vi "RTS Get Seq Index.vi"(8 "error in (no error)":errorcluster, 11 "Chamber 1-1 Input":T1[](array[typedef]) {"Start Time" format="%<%X\n%x>T"; "End Time" format="%<%X\n%x>T"}) -> (0 "Error Out":errorcluster, 1 "Times Up?":bool, 2 "Index Number":i32, 3 "Chamber 1-1 Output":T1[](array[typedef]) {"Start Time" format="%<%X\n%x>T"; "End Time" format="%<%X\n%x>T"})   [LabVIEW 2016]
uses:
  Type Definitions/RTS Door Ops Client.ctl
  Type Definitions/RTS Door Opening Schedule.ctl
  Type Definitions/RTS Door Ops Sequence.ctl
panel:
  # "Chamber Conditions:"
  # "Chamber Conditions:"
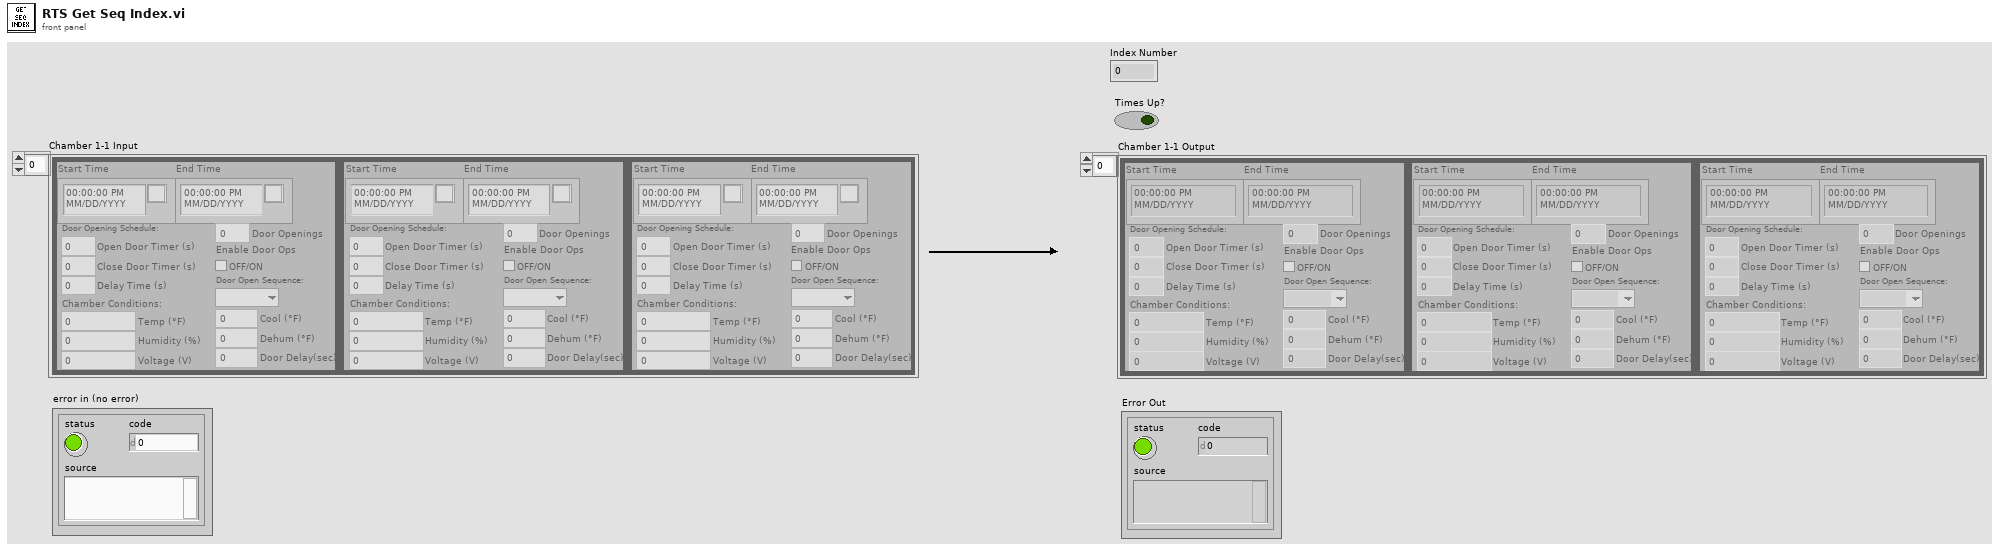
[diagram p1: front panel]
types:
  T1 = typedef "RTS Door Ops Client.ctl" = cluster{"End Time":timestamp, "Start Time":timestamp, "Door Opening Schedule:":T2, "Enable Door Ops":bool, "Door Openings":u32, "Temp (°F)":dbl, "Humidity (%)":dbl, "Voltage (V)":dbl, "Door Open Sequence:":T3, "Door Delay(sec)":dbl, "Dehum (°F)":dbl, "Cool (°F)":dbl}
  T2 = typedef "RTS Door Opening Schedule.ctl" = cluster{"Open Door Timer (s)":dbl, "Delay Time (s)":dbl, "Close Door Timer (s)":dbl}
  T3 = typedef "RTS Door Ops Sequence.ctl" = enum16{"", "1st", "2nd", "3rd"}
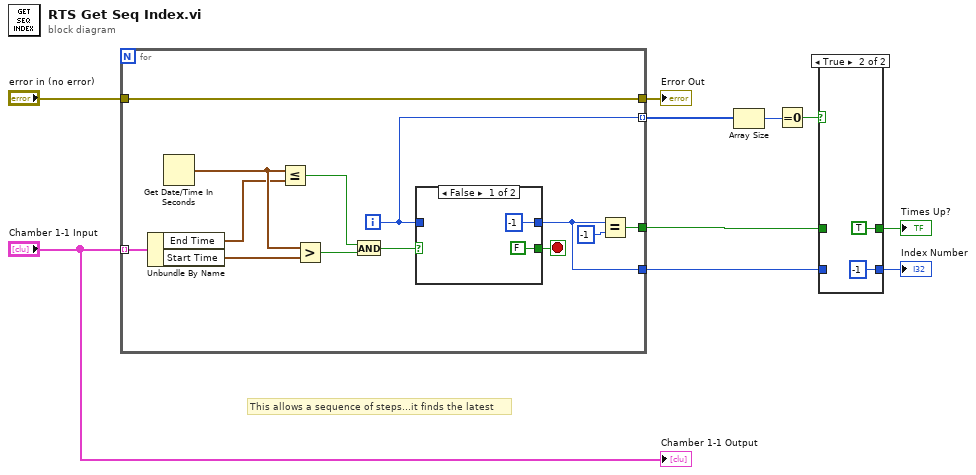
[diagram p0: block diagram]
diagram:
  # "This allows a sequence of steps...it finds the latest"
  n1 = for {
    tunnel: [w22] -> w7
    tunnel: "Chamber 1-1 Input" -> [w16] mode=indexing
    tunnel: [w13] -> w9
    tunnel: "error in (no error)" -> [w15]
    tunnel: [w15] -> w6
    tunnel: [w11] -> w5 mode=indexing
    i -> [w11]
    stop <- w12 stop-if-true
    n2 = Unbundle By Name(w16) -> ("End Time"=w14:timestamp, "Start Time"=w18:timestamp)
    n3 = Get Date/Time In Seconds() -> (seconds since 1Jan1904=w19:timestamp)
    n4 = Less Or Equal?(x=w19, y=w14) -> (x <= y?=w21:bool)
    n5 = Greater?(x=w19, y=w18) -> (0:w20:bool)
    n6 = And(x=w21, y=w20) -> (x .and. y?=w17:bool)
    n7 = case shown="False" w17 {
      selector: w17 -> [_ w26]
      tunnel: [-1 w27] -> w13
      tunnel: w11 -> [_ w27]
      tunnel: [FALSE w26] -> w12
      frame False {
      }
      frame True {
      }
    }
    n8 = Equal?(x=w13, y=-1) -> (x = y?=w22:bool)
  }
  "Error Out" <- w6
  n9 = Array Size(array=w5) -> (size(s)=w2:i32)
  n10 = Equal To 0?(x=w2) -> (x = 0?=w1:bool)
  n11 = case shown="True" w1 {
    tunnel: w9 -> [w28 _]
    tunnel: w7 -> [w29 _]
    tunnel: [w29 TRUE] -> w4
    tunnel: [w28 -1] -> w3
    frame False {
    }
    frame True {
    }
  }
  "Index Number" <- w3
  "Times Up?" <- w4
  "Chamber 1-1 Output" <- "Chamber 1-1 Input"
